vi "saveEEPFiles.vi"(10 "input_path":path, 11 "midVar_ref_readPorts":refnum<vi>[](array[refnum])=[refnum, refnum, refnum, refnum, refnum]) -> ()   [LabVIEW 2011]
uses:
  <vilib>/Utility/file.llb/Write To Spreadsheet File (string).vi
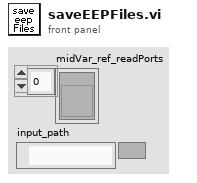
[diagram p1: front panel]
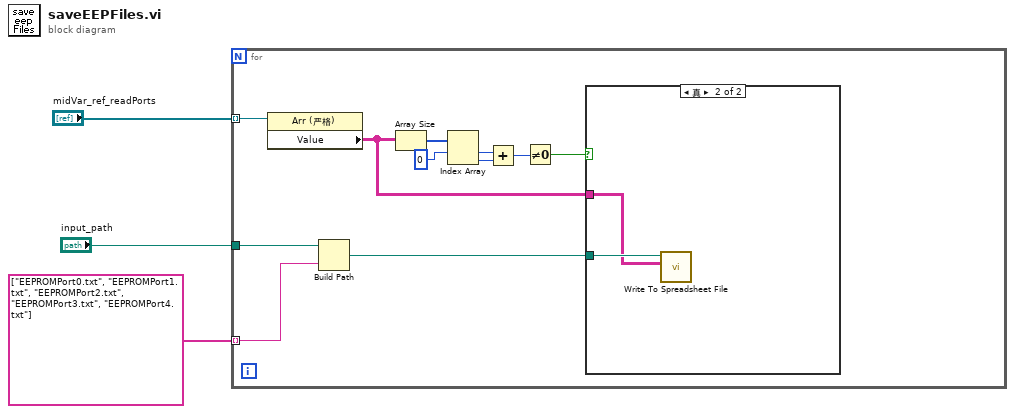
[diagram p0: block diagram]
diagram:
  n1 = for {
    tunnel: "midVar_ref_readPorts" -> [w14] mode=indexing
    tunnel: string[] ["EEPROMPort0.txt", "EEPROMPort1.txt", "EEPROMPort2.txt", "EEPROMPort3.txt", "EEPROMPort4.txt"] -> [w5] mode=indexing
    tunnel: "input_path" -> [w6]
    n2 = property class="Arr (严格)"(reference=w14) -> ("Value"=w7:string[][])  [unwired: 1 in, 2 out]
    n3 = Build Path(base path=w6, name or relative path=w5) -> (appended path=w4:path)
    n4 = Array Size(array=w7) -> (size(s)=w13:i32[])
    n5 = Index Array(array=w13, index #1=0 ("索引")) -> (element #1=w10:i32, element #2=w11:i32)  [unwired: 1 in]
    n6 = Add(x=w10, y=w11) -> (x+y=w9:i32)
    n7 = Not Equal To 0?(x=w9) -> (x != 0?=w8:bool)
    n8 = case shown="真" w8 {
      tunnel: w7 -> [_ w15]
      tunnel: w4 -> [_ w16]
      frame False {
      }
      frame True {
        n9 = call-poly <vilib>:"Write To Spreadsheet File.vi"("2D data"=w15, "file path (dialog if empty)"=w16) -> ()  [unwired: 6 in, 1 out]
      }
    }
  }
